vi "Start GNU Octave.vi"(0 "working directory":path, 1 "full start timeout [ms] (20000)":u32=20000, 5 "octave exe file or directory":path=path "C:/Octave/Octave-4.0.0/bin", 7 "path to lv_proc.dll (.)":path, 9 "hide debug console (T)":bool=TRUE, 11 "error in":errorcluster, 12 "wait for full GNU Octave start (T)":bool=TRUE) -> (3 "GNU Octave version":string, 4 "GOLPI ref. out":T1={"pipe handle"={"lv_proc.dll file path"=path "", "process instance handle"=[], "debug mode"=FALSE, "debug data"=[]}, "fast read timeout [ms]"=500, "fast read settle time [ms]"=10, "fast read to multiple [ms]"=1, "max elements per input line"=100, "slow read timeout [ms]"=500, "stdin double format specifier"="", "max elements per stdout output column"=100}, 14 "initial output":string, 15 "error out":errorcluster)   [LabVIEW 2013, in "GOLPI library.lvlib"]
doc: "Starts the GNU Octave and sets the working directory. Octave binary directory is the directory containing the 'octave.exe' executable file. Initial output is the informations printed after start on the screen by GNU Octave. Set higher vlaue for 'Full start timeout' in the case GNU Octave loads a lot of packages.\n\nIf 'Wait for full GNU Octave start' is disabled, vi starts GNU Octave and do not wait for the end of starting sequence. It is usefull if GNU Octave loads a lot of packages at startup and the start can take several seconds. 'Version' and 'Initial output' is not returned. User can check himself if Octave finished starting sequence by waiting for keyword 'GOLPImarkstart' in the stdout (i.e. use 'Read Output Till Keyword.vi').\n\nSet 'hide window' to false to show console window. Thus user can watch commands sent to GNU Octave and its output. Window is not interactive, only for debug purposes.\n\n---\nGOLPI works only with lv_proc.dll library, which is part of vipm package or should be delivered together with packed library. Placement of this dll is selected in terminal of Start GNU Octave.vi."
uses:
  GOLPI library.lvlib
  GOLPI reference Type Def.ctl
  LV Process source distribution/Pipe Handle.ctl
  Private/Type Definitions/Custom Error Codes Enum Type Def.vi
  <vilib>/regexp/Match Regular Expression.xnode
  LV Process source distribution/LV Process library.lvlib
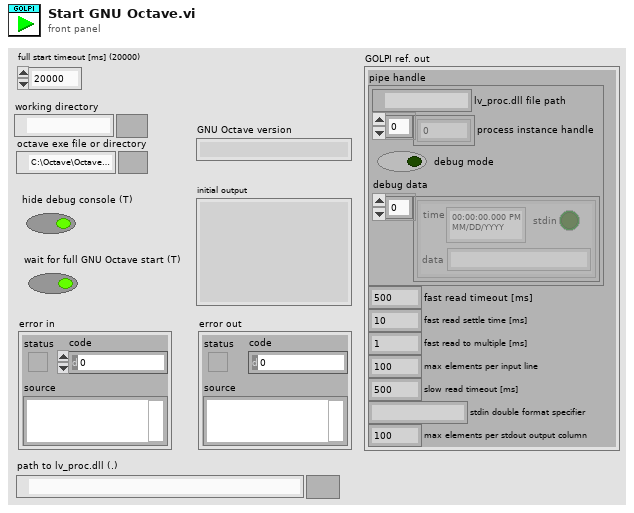
[diagram p1: front panel]
types:
  T1 = typedef "GOLPI library.lvlib/GOLPI reference Type Def.ctl" = cluster{"pipe handle":T2, "fast read timeout [ms]":u32, "fast read settle time [ms]":u32, "fast read to multiple [ms]":u32, "max elements per input line":u32, "slow read timeout [ms]":u32, "stdin double format specifier":string, "max elements per stdout output column":u32}
  T2 = typedef "LV Process library.lvlib/Pipe Handle.ctl" = cluster{"lv_proc.dll file path":path, "process instance handle":u32[], "debug mode":bool, "debug data":cluster{"time":timestamp, "stdin":bool, "data":string}[]}
  T3 = typedef "GOLPI library.lvlib/Custom Error Codes Enum Type Def.vi" = enum16{"no error", "00 working directory PAR1 missing", "01 octave binary PAR1 missing", "02 octave report error PAR1", "03 empty output last cmd PAR1", "04 missing temporary file PAR1", "05 pwd PAR 1 not exist", "10 var PAR1 not string, vect", "11 var PAR1 not num, scal, ~compl", "12 var PAR1 not num, scal, compl", "13 var PAR1 not num, vect, ~compl", "14 var PAR1 not num, vect, compl", "15 var PAR1 not num, mat, ~compl", "16 var PAR1 not num, mat, ~compl", "30 read timeout", "99 not finished"}
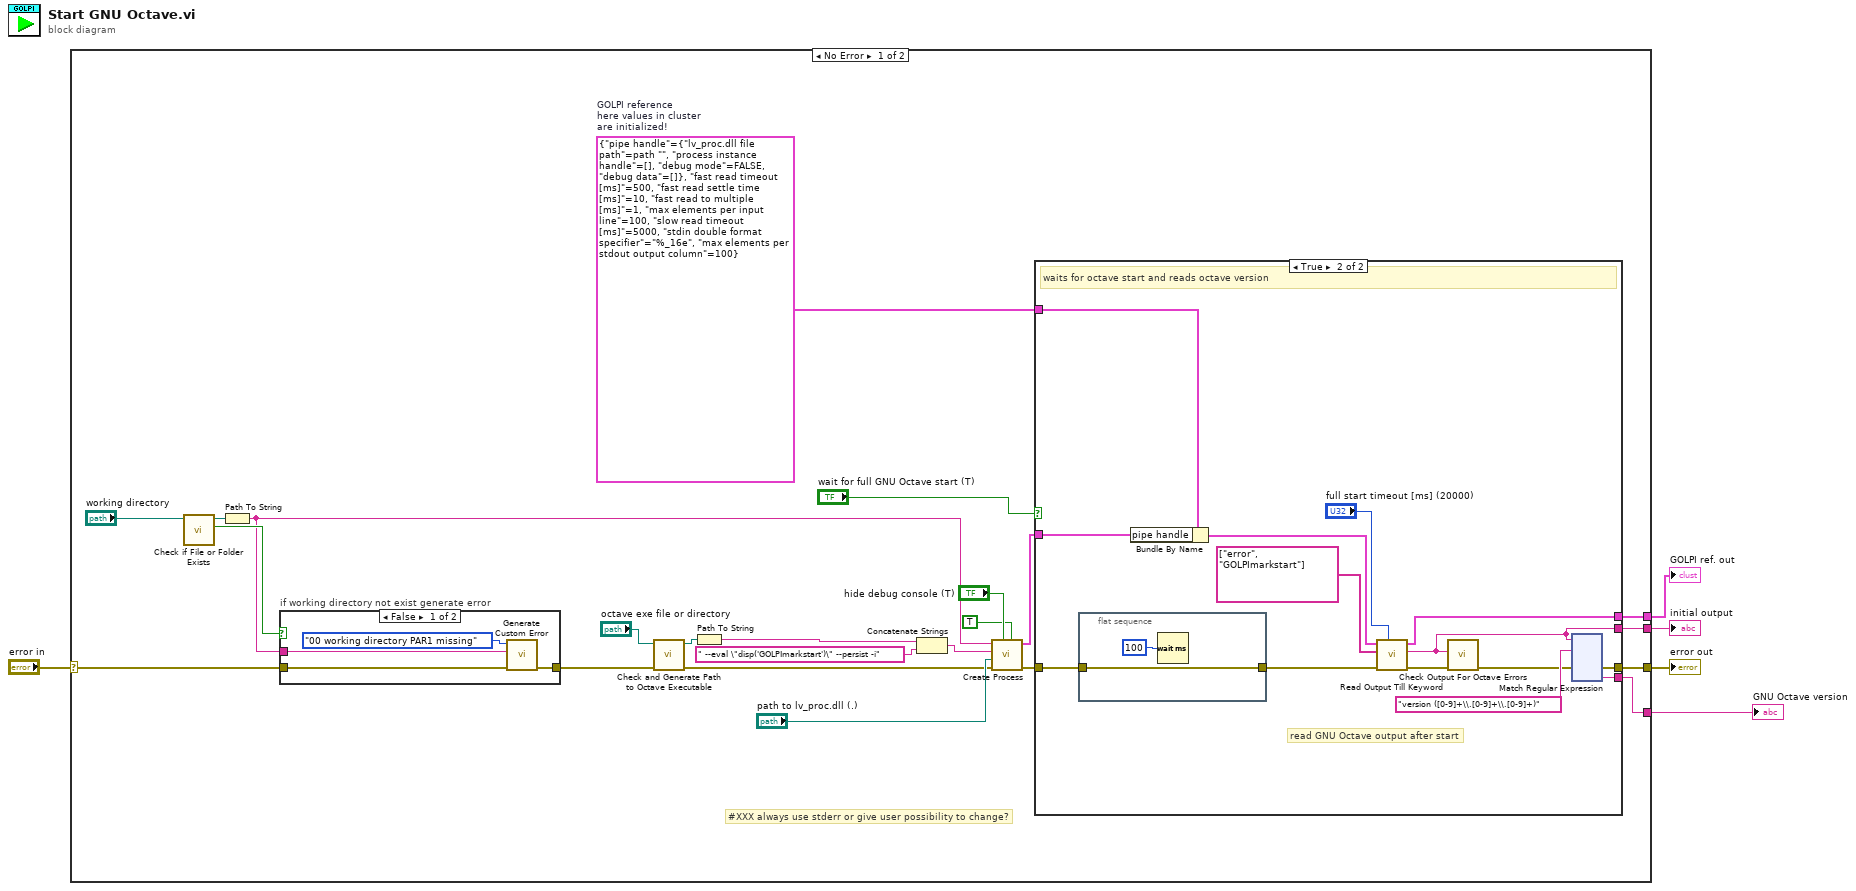
[diagram p0: block diagram]
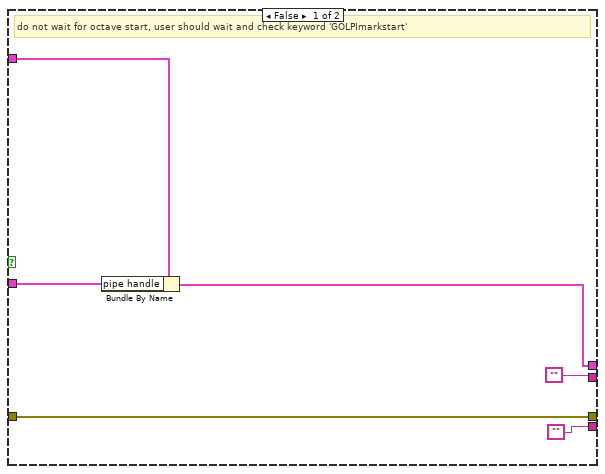
[diagram p2: hidden frame]
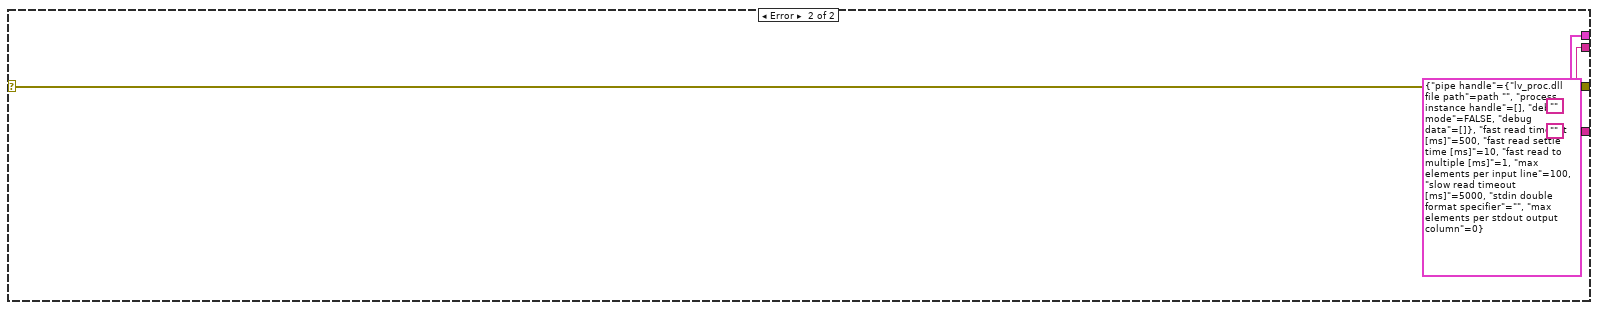
[diagram p4: hidden frame]
diagram:
  n1 = case shown="No Error" "error in" {
    selector: "error in" -> [w22 w175]
    tunnel: [w13 w175] -> w4
    tunnel: [w20 ""] -> w3
    tunnel: [w12 ""] -> w2
    tunnel: [w17 T1 {"pipe handle"={"lv_proc.dll file path"=path "", "process instance handle"=[], "debug mode"=FALSE, "debug data"=[]}, "fast read timeout [ms]"=500, "fast read settle time [ms]"=10, "fast read to multiple [ms]"=1, "max elements per input line"=100, "slow read timeout [ms]"=5000, "stdin double format specifier"="", "max elements per stdout output column"=0} ("GOLPI ref.")] -> w1
    frame No Error {
      w19 = T1 {"pipe handle"={"lv_proc.dll file path"=path "", "process instance handle"=[], "debug mode"=FALSE, "debug data"=[]}, "fast read timeout [ms]"=500, "fast read settle time [ms]"=10, "fast read to multiple [ms]"=1, "max elements per input line"=100, "slow read timeout [ms]"=5000, "stdin double format specifier"="%_16e", "max elements per stdout output column"=100}  # GOLPI reference here values in cluster are initialized!
      # "#XXX always use stderr or give user possibility to change?"
      n2 = call <vilib>:"Check if File or Folder Exists.vi"("path"="working directory") -> ("file or folder exists?"=w24:bool, "dup path"=w25:path)  [unwired: 8 in, 1 out]
      n3 = Path To String(path=w25) -> (string=w23:string)
      n4 = case "if working directory not exist generate error" shown="False" w24 {
        tunnel: [w168 w171] -> w9
        tunnel: w22 -> [w167 w171]
        tunnel: w23 -> [w170 _]
        frame False {
          n5 = call "Generate Custom Error.vi"("error in"=w167, "PAR1"=w170, "GOLPI error"=Custom_Error_Codes_Enum_Type_Def.vi."00 working directory PAR1 missing" ("Enum")) -> ("error out"=w168:errorcluster)  [unwired: 8 in]
        }
        frame True {
        }
      }
      n6 = call "Check and Generate Path to Octave Executable.vi"("error in (no error)"=w9, "octave executable file or directory with executable"="octave exe file or directory") -> ("error out"=w8:errorcluster, "path to exe"=w6:path)  [unwired: 8 in]
      n7 = Path To String(path=w6) -> (string=w16:string)
      n8 = Concatenate Strings(w16, " --eval \"disp('GOLPImarkstart')\" --persist -i" ("string")) -> (w14:string)
      n9 = call "Create Process.vi"("use stderr (F)"=TRUE, "hide window (T)"="hide debug console (T)", "error in"=w8, "path to lv_proc.dll (.)"="path to lv_proc.dll (.)", "command"=w14, "working directory"=w23) -> ("error out"=w21:errorcluster, "pipe out"=w18:T2)  [unwired: 4 in]
      n10 = case shown="True" "wait for full GNU Octave start (T)" {
        tunnel: w21 -> [w34 w48]
        tunnel: ["" w45] -> w20
        tunnel: w19 -> [w31 w44]
        tunnel: w18 -> [w30 w43]
        tunnel: [w29 w41] -> w17
        tunnel: [w34 w40] -> w13
        tunnel: ["" w36] -> w12
        frame False {
          # "do not wait for octave start, user should wait and check keyword 'GOLPImarkstart'"
          n11 = Bundle By Name(cluster=w31, "pipe handle"=w30) -> (w29:T1)
        }
        frame True {
          # "read GNU Octave output after start"
          # "waits for octave start and reads octave version"
          n12 = flat-sequence {
            tunnel: [w165] -> w47
            tunnel: w48 -> [w165]
            frame #0 {
              n13 = Wait (ms)(milliseconds to wait=u32 100) -> ()  [unwired: 1 out]
            }
          }
          n14 = Bundle By Name(cluster=w44, "pipe handle"=w43) -> (w42:T1)
          n15 = call "Read Output Till Keyword.vi"("timeout [ms]"="full start timeout [ms] (20000)", "error in"=w47, "keywords"=string[] ["error", "GOLPImarkstart"], "GOLPI ref. in"=w42) -> ("error out"=w38:errorcluster, "read buffer"=w36:string, "GOLPI ref. out"=w41:T1)  [unwired: 4 in, 1 out]
          n16 = call "Check Output For Octave Errors.vi"("error in"=w38, "read buffer"=w36) -> ("error out"=w37:errorcluster)  [unwired: 9 in]
          n17 = xnode "Match Regular Expression"("input string"=w36, "regular expression"="version ([0-9]+\\.[0-9]+\\.[0-9]+)", "error in"=w37) -> ("error out"=w40:errorcluster, "submatch 1"=w45:string)  [unwired: 3 in, 4 out]
        }
      }
    }
    frame Error {
    }
  }
  "error out" <- w4
  "GNU Octave version" <- w3
  "initial output" <- w2
  "GOLPI ref. out" <- w1
